vi "Hamamatsu_temp_monitor.vi"() -> ()   [LabVIEW 2013, in "Hamamatsu_C9100-13.lvclass"]
uses:
  Hamamatsu_C9100-13.lvclass
  <vilib>/Platform/TimedLoop/XDataNode/timing_clust.ctl
  <vilib>/Platform/TimedLoop/XDataNode/nitl_modes.ctl
  <vilib>/Platform/TimedLoop/XDataNode/wakeup.ctl
  <vilib>/platform/TimedLoop/XDataNode/XDataNode.xnode
  <vilib>/Platform/TimedLoop/XDataNode/XDNodeRunTimeDep.lvlib
panel:
  out "Camera Temperature":dbl format="%.3g"
  out "error out":errorcluster
  in  "error in (no error)":errorcluster
  in  "stop":bool
  out "Waveform Chart":waveform(dbl)(graph)
  in  "Hamamatsu_C9100-13.lvclass":refnum<class "Hamamatsu_C9100-13.lvclass">
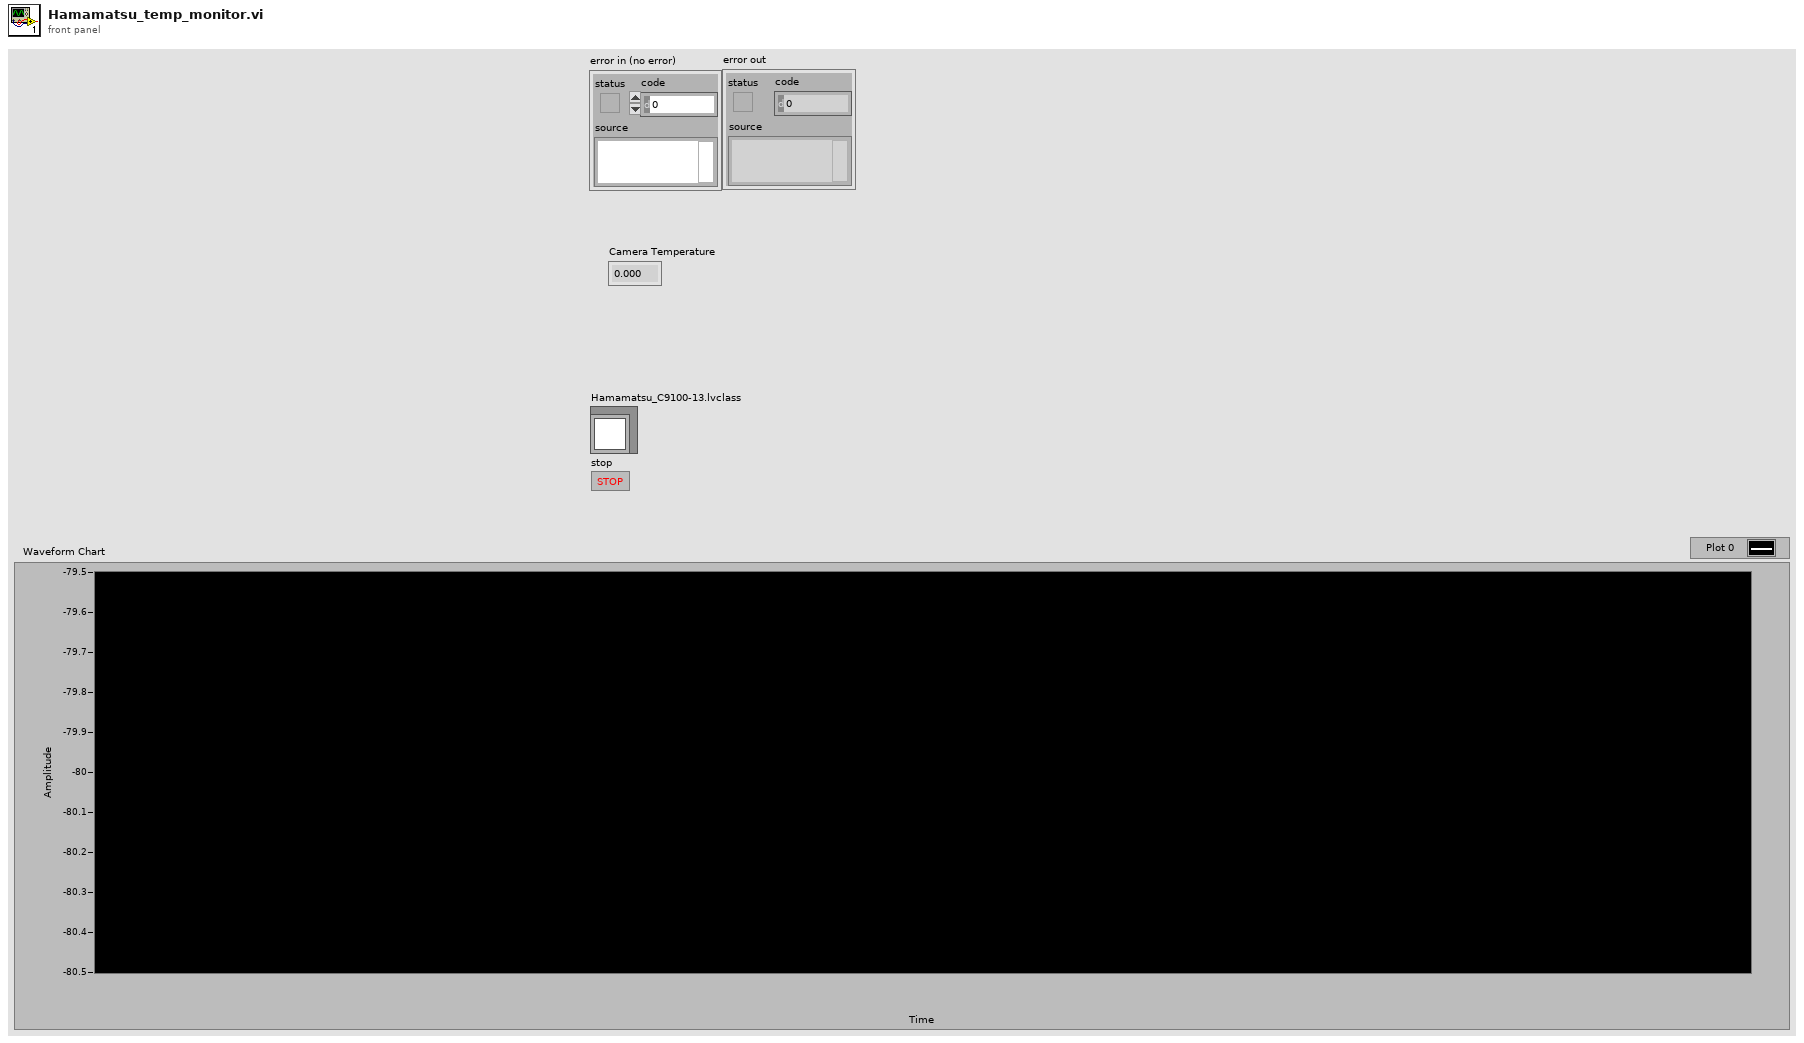
[diagram p1: front panel]
types:
  T1 = typedef "XDNodeRunTimeDep.lvlib/timing_clust.ctl" = cluster{"Expected End [f-1]":u64, "Actual End [f-1]":u64, "Finished Late? [f-1]":bool, "Expected End [i-1]":u64, "Actual End [i-1]":u64, "Finished Late? [i-1]":bool, "Expected Start [i]":u64, "Actual Start [i]":u64, "Expected Start [f]":u64, "Actual Start [f]":u64, "Source Name":string, "Structure Name":string, "Period":i64, "Deadline":i64, "Offset":i64, "Start":i64, "Priority":i32, "Timeout":i32, "Mode":T2, "Wakeup Reason":T3, "Error":errorcluster, "Source Type":string, "Secondary Source Type":string, "Global End Time":u64, "Global Start Time":u64, "Frame Duration":u64, "Iteration Duration":u64, "Assigned CPU":i32, "I/O Scan Engine Mode":u32}
  T2 = typedef "XDNodeRunTimeDep.lvlib/nitl_modes.ctl" = enum32{"No Change", "Process missed periods, maintain original phase", "Discard missed periods, maintain original phase", "Process missed periods, ignore original phase", "Discard missed periods, ignore original phase"}
  T3 = typedef "XDNodeRunTimeDep.lvlib/wakeup.ctl" = enum32{"Normal", "Aborted", "Asynchronous wakeup", "Timing source error", "Timed loop error", "Timeout"}
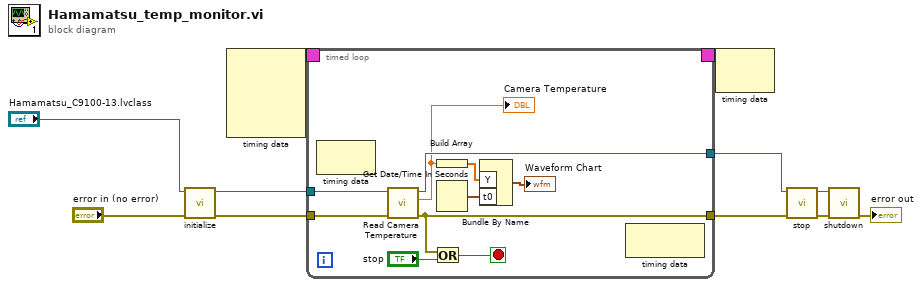
[diagram p0: block diagram]
diagram:
  n1 = call-dynamic "initialize.vi"("error in (no error)"="error in (no error)", "Hamamatsu_C9100-13 in"="Hamamatsu_C9100-13.lvclass") -> ("error out"=w9:errorcluster, "Hamamatsu_C9100-13 out"=w10:refnum<class "Hamamatsu_C9100-13.lvclass">)  [unwired: 8 in]
  n2 = node-c288() -> (w8:T1)  [unwired: 4 in]
  n3 = timed-loop {
    tunnel: w10 -> [w21]
    tunnel: w9 -> [w20]
    timing: w8 -> [_]
    timing-out: [_] -> w7
    tunnel: [w17] -> w6
    tunnel: [w16] -> w5
    stop <- w18 stop-if-true
    n4 = node-c288() -> ()  [unwired: 1 in, 1 out]
    n5 = call-dynamic "Read Camera Temperature.vi"("error in (no error)"=w20, "Hamamatsu_C9100-13 in"=w21) -> ("error out"=w16:errorcluster, "Camera Temperature"=w13:dbl, "Hamamatsu_C9100-13 out"=w17:refnum<class "Hamamatsu_C9100-13.lvclass">)  [unwired: 7 in]
    "Camera Temperature" <- w13
    n6 = Or(x=w16, y="stop") -> (x .or. y?=w18:bool)
    n7 = Build Array(w13) -> (w15:dbl[])
    n8 = Get Date/Time In Seconds() -> (seconds since 1Jan1904=w14:timestamp)
    n9 = Bundle By Name("Y"=w15, "t0"=w14) -> (→"Waveform Chart":waveform(dbl))  [unwired: 1 in]
    n10 = node-c288() -> ()  [unwired: 1 in, 1 out]
  }
  n11 = node-c288(w7) -> ()  [unwired: 1 out]
  n12 = call-dynamic "stop.vi"("error in (no error)"=w5, "Hamamatsu_C9100-13 in"=w6) -> ("error out"=w4:errorcluster, "Hamamatsu_C9100-13 out"=w1:refnum<class "Hamamatsu_C9100-13.lvclass">)  [unwired: 8 in]
  n13 = call-dynamic "shutdown.vi"("error in (no error)"=w4, "Hamamatsu_C9100-13 in"=w1) -> ("error out"=→"error out":errorcluster)  [unwired: 8 in, 1 out]
